vi "Create Seq URL.vi"(8 "error in (no error)":errorcluster, 10 "Path":string, 11 "Sequencing Control in":refnum<class "Sequencing Control.lvclass">) -> (0 "error out":errorcluster, 2 "Request URL":string, 3 "Sequencing Control out":refnum<class "Sequencing Control.lvclass">)   [LabVIEW 2020, in "VolatusSeqGUI.lvlib" / "Sequencing Control.lvclass"]
uses:
  Sequencing Control.lvclass
  Sequencing Control.lvclass/Sequencing Control.ctl
  Volatus/VolatusAPI/VolatusAPI.lvclass
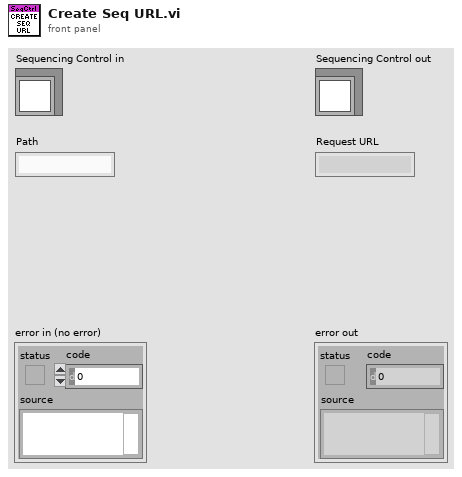
[diagram p1: front panel]
types:
  T1 = typedef "VolatusSeqGUI.lvlib/Sequencing Control.lvclass/Sequencing Task.ctl" = cluster{"Node":string, "Task":string}
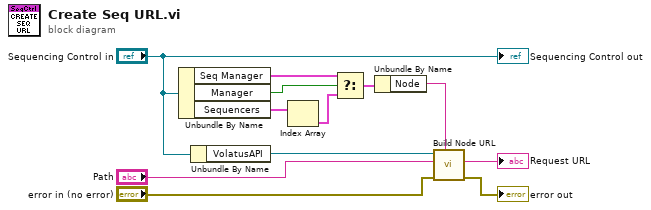
[diagram p0: block diagram]
diagram:
  n1 = Unbundle By Name("Sequencing Control in") -> ("Seq Manager"=w10:T1, "Manager"=w9:bool, "Sequencers"=w12:T1[])
  n2 = Unbundle By Name("Sequencing Control in") -> ("VolatusAPI"=w8:refnum<class "VolatusAPI.lvclass">)
  n3 = Index Array(array=w12) -> (element=w11:T1)  [unwired: 1 in]
  n4 = Select(t=w10, s=w9, f=w11) -> (s? t:f=w7:T1)
  n5 = Unbundle By Name(w7) -> ("Node"=w6:string)
  n6 = call "Build Node URL.vi"("Node Name"=w6, "error in (no error)"="error in (no error)", "Path"="Path", "VolatusAPI in"=w8) -> ("error out"=→"error out":errorcluster, "Request URL"=→"Request URL":string)  [unwired: 5 in, 1 out]
  "Sequencing Control out" <- "Sequencing Control in"
